vi "TimeDate String to Timestamp.vi"(11 "Time/Date String":string="04/04/2012  09:59.55.18") -> (3 "Timestamp":timestamp)   [LabVIEW 2023]
uses:
  <vilib>/Utility/miscctls.llb/LVDateTimeRec.ctl
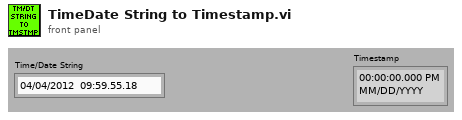
[diagram p1: front panel]
types:
  T1 = typedef "LVDateTimeRec.ctl" = cluster{"fractional second":dbl, "second":i32, "minute":i32, "hour":i32, "day of month":i32, "month":i32, "year":i32, "day of week":i32, "day of year":i32, "DST":i32}
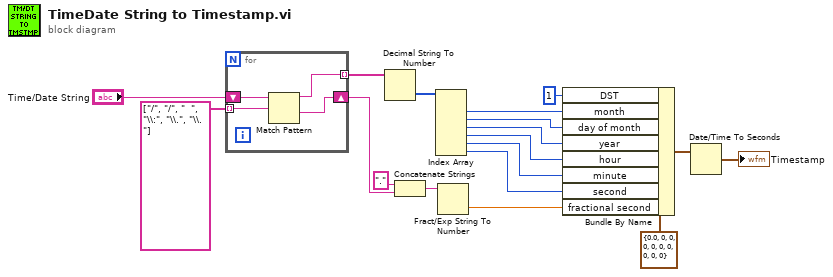
[diagram p0: block diagram]
diagram:
  n1 = for {
    shift-right: [w21] -> w7
    shift-left: "Time/Date String" -> [w22]
    tunnel: [w20] -> w14 mode=indexing
    tunnel: string[] ["/", "/", "  ", "\\:", "\\.", "\\."] -> [w19] mode=indexing
    n2 = Match Pattern(string=w22, regular expression=w19) -> (before substring=w20:string, after substring=w21:string)  [unwired: 1 in, 2 out]
  }
  n3 = Decimal String To Number(string=w14) -> (number=w13:i32[])  [unwired: 2 in, 1 out]
  n4 = Concatenate Strings("." ("string"), w7) -> (w4:string)
  n5 = Index Array(array=w13) -> (element #1=w12:i32, element #2=w11:i32, element #3=w10:i32, element #4=w9:i32, element #5=w8:i32, element #6=w1:i32)  [unwired: 6 in]
  n6 = Fract/Exp String To Number(string=w4) -> (number=w2:dbl)  [unwired: 3 in, 1 out]
  n7 = Bundle By Name(cluster=T1 {"fractional second"=0.0, "second"=0, "minute"=0, "hour"=0, "day of month"=0, "month"=0, "year"=0, "day of week"=0, "day of year"=0, "DST"=0} ("date time rec"), "DST"=1, "month"=w12, "day of month"=w11, "year"=w10, "hour"=w9, "minute"=w8, "second"=w1, "fractional second"=w2) -> (w16:T1)
  n8 = Date/Time To Seconds(2:w16) -> (0:→"Timestamp":timestamp)  [unwired: 1 in]
